vi "MIMO_LOOPBACK.vi"() -> ()   [LabVIEW 2012]
panel:
  in  "Chanel config":T1={"Port 1 -> Port 1"={"Atenuation [dB]"=6.0, "Noise Std. Dev."=0.01, "Initial phase [deg]"=125.0, "Freq. Shift [Hz/Hz]"=0.001}, "Port 1 -> Port 2"={"Atenuation [dB]"=9.0, "Noise Std. Dev."=0.01, "Initial phase [deg]"=125.0, "Freq. Shift [Hz/Hz]"=0.001}, "Port 2 -> Port 1"={"Atenuation [dB]"=9.0, "Noise Std. Dev."=0.01, "Initial phase [deg]"=125.0, "Freq. Shift [Hz/Hz]"=0.001}, "Port 2 -> Port 2"={"Atenuation [dB]"=3.0, "Noise Std. Dev."=0.01, "Initial phase [deg]"=125.0, "Freq. Shift [Hz/Hz]"=0.001}} {"Port 2 -> Port 2"."Freq. Shift [Hz/Hz]" min=0.0 max=1.0 step=0.0001 format="%0.4f"; "Port 2 -> Port 2"."Noise Std. Dev." format="%0.2f"; "Port 2 -> Port 2"."Atenuation [dB]" format="%0.2f"; "Port 2 -> Port 1"."Freq. Shift [Hz/Hz]" min=0.0 max=1.0 step=0.0001 format="%0.4f"; "Port 2 -> Port 1"."Noise Std. Dev." format="%0.2f"; "Port 2 -> Port 1"."Atenuation [dB]" format="%0.2f"; "Port 1 -> Port 2"."Freq. Shift [Hz/Hz]" min=0.0 max=1.0 step=0.0001 format="%0.4f"; "Port 1 -> Port 2"."Noise Std. Dev." format="%0.2f"; "Port 1 -> Port 2"."Atenuation [dB]" format="%0.2f"; "Port 1 -> Port 1"."Freq. Shift [Hz/Hz]" min=0.0 max=1.0 step=0.0001 format="%0.4f"; "Port 1 -> Port 1"."Noise Std. Dev." format="%0.2f"; "Port 1 -> Port 1"."Atenuation [dB]" format="%0.2f"}
  in  "System options":T2={"Samples per symbol"=6, "Roll-Off"=0.75, "Filter length (symbols)"=3, "Modulation Type"=enum."16-QAM", "Payload Symbols"=1008, "Symbols per Pilot"=6} {"Symbols per Pilot" min=6 max=16 step=2; "Payload Symbols" min=16 max=8192 step=16; "Filter length (symbols)" min=1 max=9 step=2; "Roll-Off" min=0.0 max=1.0 step=0.01; "Samples per symbol" min=2 max=32 step=2}
  out "Constellation":cluster{dbl[], dbl[]}[](graph)
  out "Rx data":string[](array[string])=["The quick brown fox jumps over the lazy dog", "El veloz murciélago hindú comía feliz cardillo y kiwi", "Jove xef, porti whisky amb quinze glaçons d'hidrogen, coi!", ""]
  out "Link occupation [%]":dbl(knob)=52.57936507936508 scale=0.0..100.0
  in  "Tx data":string[](array[string])=["The quick brown fox jumps over the lazy dog", "El veloz murciélago hindú comía feliz cardillo y kiwi", "Jove xef, porti whisky amb quinze glaçons d'hidrogen, coi!"]
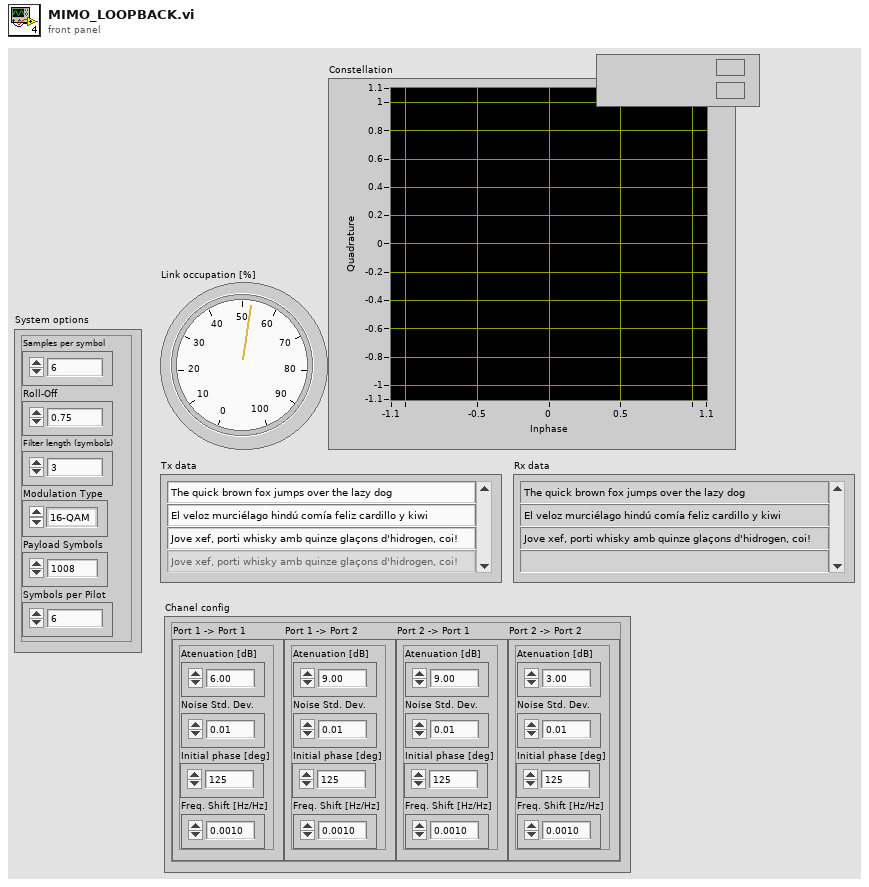
[diagram p1: front panel]
types:
  T1 = cluster{"Port 1 -> Port 1":cluster{"Atenuation [dB]":dbl, "Noise Std. Dev.":dbl, "Initial phase [deg]":dbl, "Freq. Shift [Hz/Hz]":dbl}, "Port 1 -> Port 2":cluster{"Atenuation [dB]":dbl, "Noise Std. Dev.":dbl, "Initial phase [deg]":dbl, "Freq. Shift [Hz/Hz]":dbl}, "Port 2 -> Port 1":cluster{"Atenuation [dB]":dbl, "Noise Std. Dev.":dbl, "Initial phase [deg]":dbl, "Freq. Shift [Hz/Hz]":dbl}, "Port 2 -> Port 2":cluster{"Atenuation [dB]":dbl, "Noise Std. Dev.":dbl, "Initial phase [deg]":dbl, "Freq. Shift [Hz/Hz]":dbl}}
  T2 = cluster{"Samples per symbol":i32, "Roll-Off":dbl, "Filter length (symbols)":i32, "Modulation Type":enum16{"BPSK", "4-QAM", "16-QAM", "64-QAM"}, "Payload Symbols":i32, "Symbols per Pilot":i32}
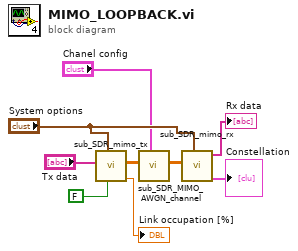
[diagram p0: block diagram]
diagram:
  n1 = call "sub_SDR_mimo_tx.vi"("Init Tx Buffer"=FALSE, "System options"="System options", "Packets"="Tx data") -> ("Link occupation [%]"=→"Link occupation [%]":dbl, "Tx Frame"=w2:cdb[][])  [unwired: 5 in, 2 out]
  n2 = call "sub_SDR_MIMO_AWGN_channel.vi"("Chanel config"="Chanel config", "Channel in"=w2) -> ("Channel Out"=w3:cdb[][])  [unwired: 9 in]
  n3 = call "sub_SDR_mimo_rx.vi"("System options"="System options", "Radio Frame"=w3) -> ("Constellation Data"=→"Constellation":cluster{dbl[], dbl[]}[], "Received Packets in current frame"=→"Rx data":string[])  [unwired: 5 in, 3 out]
